vi "compare.vi"() -> ()   [LabVIEW 2019]
panel:
  in  "stop":bool
  out "Boolean":bool
  in  "Numeric 2":dbl
  in  "Numeric":dbl
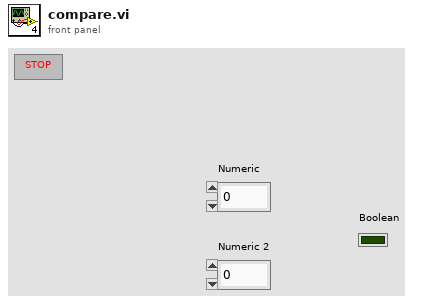
[diagram p1: front panel]
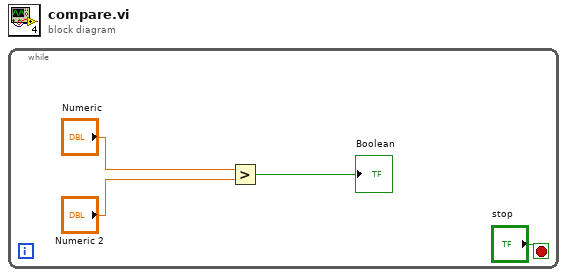
[diagram p0: block diagram]
diagram:
  n1 = while {
    stop <- "stop" stop-if-true
    n2 = Greater?(x="Numeric", y="Numeric 2") -> (0:→"Boolean":bool)
  }
